vi "OpenDevice.vi"(8 "错误输入（无错误）":errorcluster, 11 "设备类型":u32(ring)=3 items=["PCI5121"=1, "PCI9810"=2, "USBCAN1"=3, "USBCAN2"=4, "PCI9820"=5, "PCI5110"=7, "PC104CAN"=11, "CANETUDP"=12, "PCI9840B"=14, "PC104C2"=15, "PCI9820I"=16, "CANETTCP"=17, "PCIE9221"=24, "PCI5010U"=19, "USBCAN_E_U"=20, "USBCAN_2E_U"=21, "PCI5020U"=22]) -> (0 "错误输出":errorcluster, 2 "Result":bool, 3 "DevType":u32)   [LabVIEW 2013]
uses:
  ControlCAN.dll
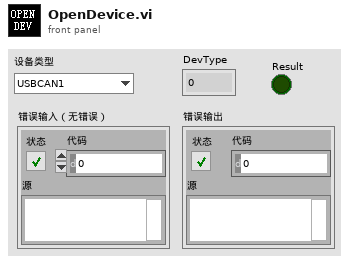
[diagram p1: front panel]
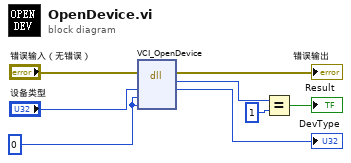
[diagram p0: block diagram]
diagram:
  w3 = u32 0 ("Reserved")
  n1 = dll-call lib="PTH1Aabs F吉利吉利CAN模拟器CAN_ZLGCANControlCAN.dll" fn="VCI_OpenDevice"(error in="错误输入（无错误）", "DevType"="设备类型", "DevIndex"=w3, "Reserved"=w3) -> (error out=→"错误输出":errorcluster, "返回类型"=w8:u32, "DevType"=→"DevType":u32)  [unwired: 4 in, 1 out]
  n2 = Equal?(x=w8, y=u32 1) -> (x = y?=→"Result":bool)
